vi "项目名称.vi"() -> ()   [LabVIEW 2013]
panel:
  in  "项目名称":string
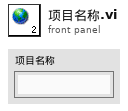
[diagram p1: front panel]
diagram:
